vi "dvp Vi Get Packet Size Sel Detail.vi"(7 "pIndex":i32, 9 "pPacketSizeSelDetailString":string, 10 "PacketSizeSel":u32, 11 "handle":u32) -> (1 "pPacketSizeSelDetailString out":string, 3 "function return":u32(ring), 5 "pIndex out":i32)   [LabVIEW 2018, in "LabViewDVPCamera.lvlib"]
doc: "LabviewDvp2Api dvpStatus dvpViGetPacketSizeSelDetail(dvpHandle handle, dvpUint32 PacketSizeSel, char* pPacketSizeSelDetailString, dvpInt32 *pIndex);"
uses:
  LabViewDVPCamera.lvlib
  LabViewDVPCamera/LabViewDVPCamera.dll
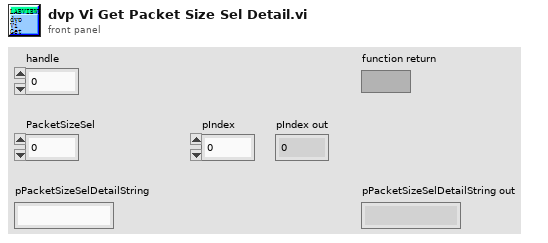
[diagram p1: front panel]
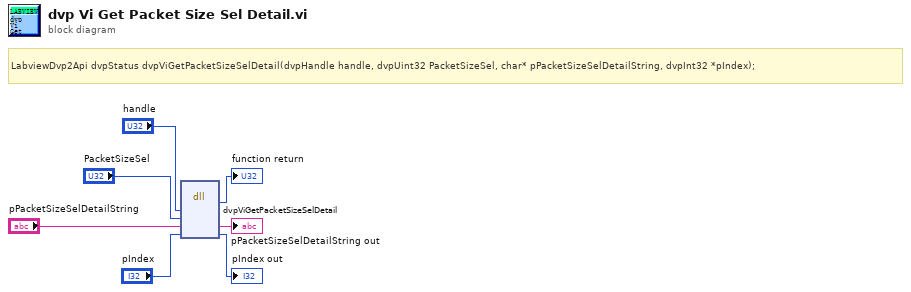
[diagram p0: block diagram]
diagram:
  # "LabviewDvp2Api dvpStatus dvpViGetPacketSizeSelDetail(dvpHandle handle, dvpUint32 PacketSizeSel, char* pPacketSizeSelDetailString, dvpInt32 *pIndex);"
  n1 = dll-call lib="C:/Program Files (x86)/DVP2 Labview cn 64/Sample/LabViewDVPCamera/LabViewDVPCamera.*" fn="dvpViGetPacketSizeSelDetail"("handle"="handle", "PacketSizeSel"="PacketSizeSel", "pPacketSizeSelDetailString"="pPacketSizeSelDetailString", "pIndex"="pIndex") -> (→"function return":u32, "pPacketSizeSelDetailString"=→"pPacketSizeSelDetailString out":string, "pIndex"=→"pIndex out":i32)  [unwired: 5 in, 2 out]
